vi "NetComm_CAN_Receive.vi"(8 "error in (no error)":errorcluster, 9 "Message ID Mask":u32=4294967295 format="%.0x", 10 "Message ID":u32 format="%.0x") -> (0 "error out":errorcluster, 1 "Data":u8[](array[numeric]), 2 "Message ID Out":u32 format="%.0x", 4 "timeStamp":u32)   [LabVIEW 2017]
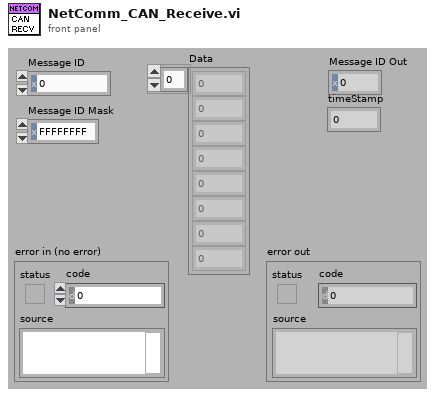
[diagram p1: front panel]
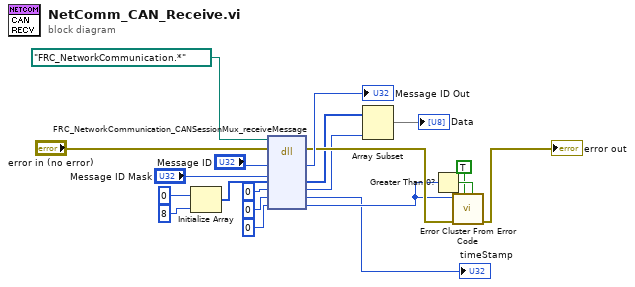
[diagram p0: block diagram]
diagram:
  n1 = Initialize Array(u8 0 ("dataSize"), 8 ("dimension size")) -> (w12:u8[])
  n2 = dll-call lib="FRC_NetworkCommunication.*" fn="FRC_NetworkCommunication_CANSessionMux_receiveMessage"(path in=path "FRC_NetworkCommunication.*", error in="error in (no error)", "messageID"="Message ID", "messageIDMask"="Message ID Mask", "data"=w12, "dataSize"=u8 0, "timeStamp"=u32 0, "status"=0) -> (error out=w11:errorcluster, "messageID"=→"Message ID Out":u32, "data"=w6:u8[], "dataSize"=w7:u8, "timeStamp"=→"timeStamp":u32, "status"=w9:i32)  [unwired: 3 in, 1 out]
  n3 = Array Subset(array=w6, length=w7) -> (→"Data":u8[])  [unwired: 1 in]
  n4 = Greater Than 0?(x=w9) -> (x > 0?=w10:bool)
  n5 = call <vilib>:"Error Cluster From Error Code.vi"("is warning? (False)"=w10, "show call chain? (False)"=TRUE, "error in (no error)"=w11, "error code (0)"=w9) -> ("error out"=→"error out":errorcluster)  [unwired: 5 out]
